vi "Test.vi"() -> ()   [LabVIEW 2014]
doc: "This VI is called when test mode begins, and will automatically be terminated when it ends. You can add manual or automatic tests and invoke them from the dashboard."
uses:
  Robot Global Data.vi
panel:
  out "Boolean":bool=TRUE
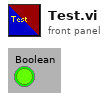
[diagram p1: front panel]
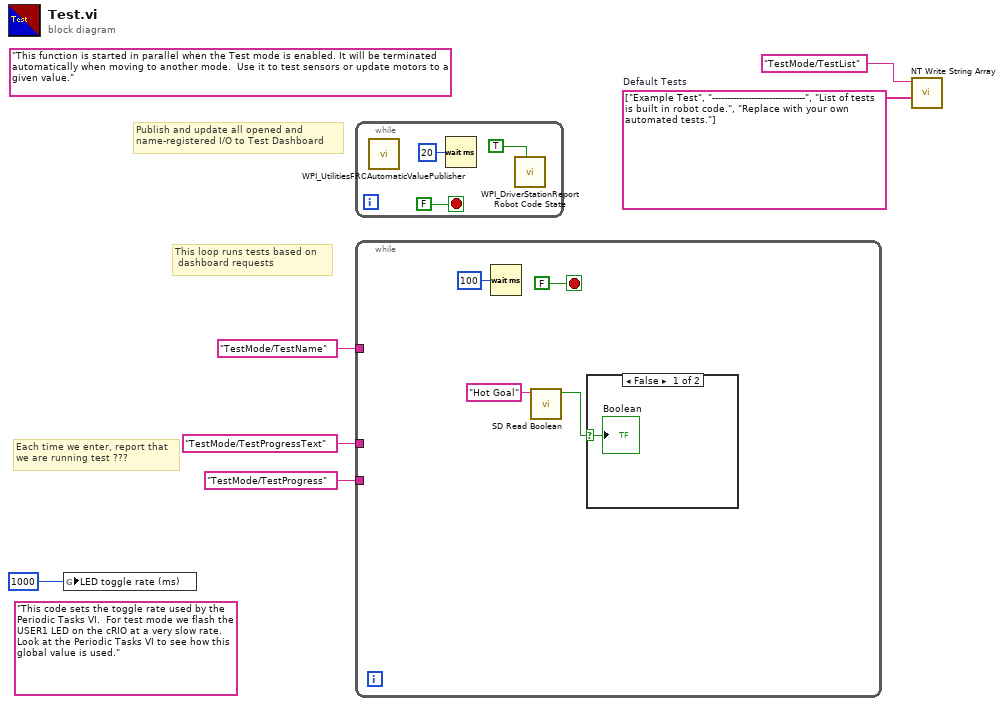
[diagram p0: block diagram]
diagram:
  w2 = string[] ["Example Test", "-------------------------------", "List of tests is built in robot code.", "Replace with your own automated tests."]  # Default Tests
  (unwired) "This code sets the toggle rate used by the Periodic Tasks VI.  For test mode we flash the USER1 LED on the cRIO at a very slow rate.  Look at the Periodic Tasks VI to see how this global value is used."
  (unwired) "This function is started in parallel when the Test mode is enabled. It will be terminated automatically when moving to another mode.  Use it to test sensors or update motors to a given value."
  # "This loop runs tests based on \n dashboard requests"
  # "Publish and update all opened and\nname-registered I/O to Test Dashboard"
  # "Each time we enter, report that\nwe are running test ???"
  n1 = global write "Robot Global Data.vi" "LED toggle rate (ms)"(u32 1000 ("LED ms toggle rate")) -> ()
  n2 = while {
    stop <- FALSE stop-if-true
    n3 = call <vilib>:"WPI_UtilitiesFRCAutomaticValuePublisher.vi"() -> ()  [unwired: 12 in]
    n4 = Wait (ms)(milliseconds to wait=u32 20) -> ()  [unwired: 1 out]
    n5 = call <vilib>:"WPI_DriverStationReport Robot Code State.vi"("Test"=TRUE ("Autonomous")) -> ()  [unwired: 10 in, 1 out]
  }
  n6 = while {
    tunnel: "TestMode/TestName" ("Name") -> [_]
    tunnel: "TestMode/TestProgressText" ("Name") -> [_]
    tunnel: "TestMode/TestProgress" ("Name") -> [_]
    stop <- FALSE stop-if-true
    n7 = Wait (ms)(milliseconds to wait=u32 100) -> ()  [unwired: 1 out]
    n8 = call <vilib>:"SD Read Boolean.vi"("Name"="Hot Goal") -> ("Boolean"=w10:bool)  [unwired: 8 in, 2 out]
    n9 = case shown="False" w10 {
      selector: w10 -> [w14 _]
      frame False {
        "Boolean" <- w14
      }
      frame True {
      }
    }
  }
  n10 = call <vilib>:"NT Write String Array.vi"("String Array"=w2, "Name"="TestMode/TestList") -> ()  [unwired: 9 in, 1 out]
